vi "Get Coverage for VIs in set.vi"(8 "error in (no error)":errorcluster, 10 "VIs":set{path}(c389), 11 "Coverage Analyzer in":refnum<class "Coverage Analyzer.lvclass">) -> (0 "error out":errorcluster, 2 "Code Coverage":map{path, dbl}(c390), 3 "Coverage Analyzer out":refnum<class "Coverage Analyzer.lvclass">)   [LabVIEW 2020, in "Coverage Analyzer.lvlib" / "Coverage Analyzer.lvclass"]
uses:
  Coverage Analyzer.lvclass
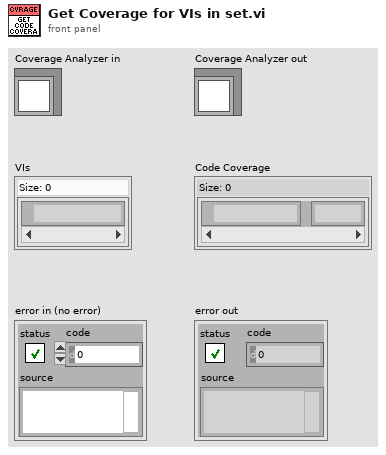
[diagram p1: front panel]
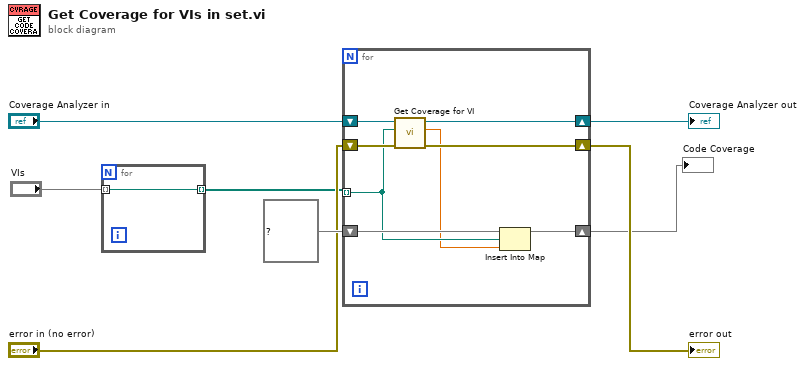
[diagram p0: block diagram]
diagram:
  n1 = for {
    tunnel: "VIs" -> [w9] mode=indexing
    tunnel: [w9] -> w1 mode=indexing
  }
  n2 = for {
    shift-right: [w16] -> w8
    shift-left: "Coverage Analyzer in" -> [w17]
    shift-right: [w14] -> w7
    shift-left: "error in (no error)" -> [w15]
    tunnel: w1 -> [w11] mode=indexing
    shift-right: [w12] -> w5
    shift-left: map{path, dbl} {} ("Code Coverage") -> [w13]
    n3 = call "Get Coverage for VI.vi"("error in (no error)"=w15, "VI Path"=w11, "Coverage Analyzer in"=w17) -> ("error out"=w14:errorcluster, "Percentage"=w10:dbl, "Coverage Analyzer out"=w16:refnum<class "Coverage Analyzer.lvclass">)  [unwired: 5 in, 1 out]
    n4 = Insert Into Map(map in=w13, key=w11, value=w10) -> (map out=w12:map{path, dbl})  [unwired: 2 out]
  }
  "error out" <- w7
  "Coverage Analyzer out" <- w8
  "Code Coverage" <- w5
